vi "Main.vi"(10 "JQMHStartup":refnum<class "RQMHStartup.lvclass">, 11 "NewTemplate in":refnum<class "CRON.lvclass">) -> ()   [LabVIEW 2024, in "CRON.lvclass"]
uses:
  CRON.lvclass
  C:/DevOps/CORTEX/JQMH/RQMHCore/ModuleCore/RQMHModule.lvclass
  RQMHCore/Startup/RQMHStartup.lvclass
  <vilib>/LabVIEW Open Source Project/Cron Scheduler/Cron/Cron.lvclass
  RQMHCore/ModQueue/RQMHMessageQueue.lvclass/RQMHMessageQueue.ctl
  RQMHCore/ModuleCore/InitialiseReplyArgs.ctl
  <vilib>/Utility/miscctls.llb/LVPointTypeDef.ctl
  RQMHCore/ModuleCore/RQMHModule.lvclass/RQMHModule.ctl
  Do Something ReplyArgs.ctl
  Do Something Args.ctl
  RQMHCore/ModuleCore/Read ModuleName.vi
  RQMHCore/ModuleCore/Read External Start.vi
  RQMHCore/ModQueue/Delacor_lib_QMH_Enqueue Message (Single).vi
  RQMHCore/ModQueue/RQMHMessageQueue.lvclass
  RQMHCore/ModuleCore/RQMHModule.lvclass
  RQMHCore/Shared/RQMHShared.lvlib
  <vilib>/LabVIEW Open Source Project/Cron Scheduler/openCron.lvlib
panel:
  out "error out":errorcluster
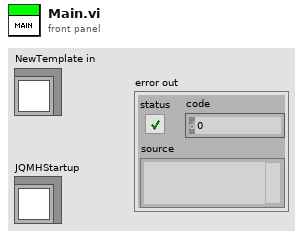
[diagram p1: front panel]
types:
  T1 = typedef "CRON.lvclass/Request Events--cluster.ctl" = cluster{"Do Something":refnum<user-event>, "Set Schedule":refnum<user-event>, "Arm":refnum<user-event>}
  T2 = cluster{"Stop Module":refnum<user-event>, "Requests":T1}
  T3 = typedef "LVPointTypeDef.ctl" = cluster{"Horizontal":i16, "Vertical":i16}
  T4 = enum32{"Invalid", "Standard", "Closed", "Hidden", "Minimized", "Maximized"}
  T5 = typedef "RQMHModule.lvclass/InitialiseReplyArgs.ctl" = cluster{"Did Init?":bool}
  T6 = typedef "CRON.lvclass/Do Something Args.ctl" = cluster{"Msg":string}
  T7 = typedef "CRON.lvclass/Do Something ReplyArgs.ctl" = cluster{"Value":dbl, "Boolean":bool}
  T8 = typedef "RQMHModule.lvclass/Reply.ctl" = cluster{"Expects Reply":bool, "Reply":refnum<notifier>}
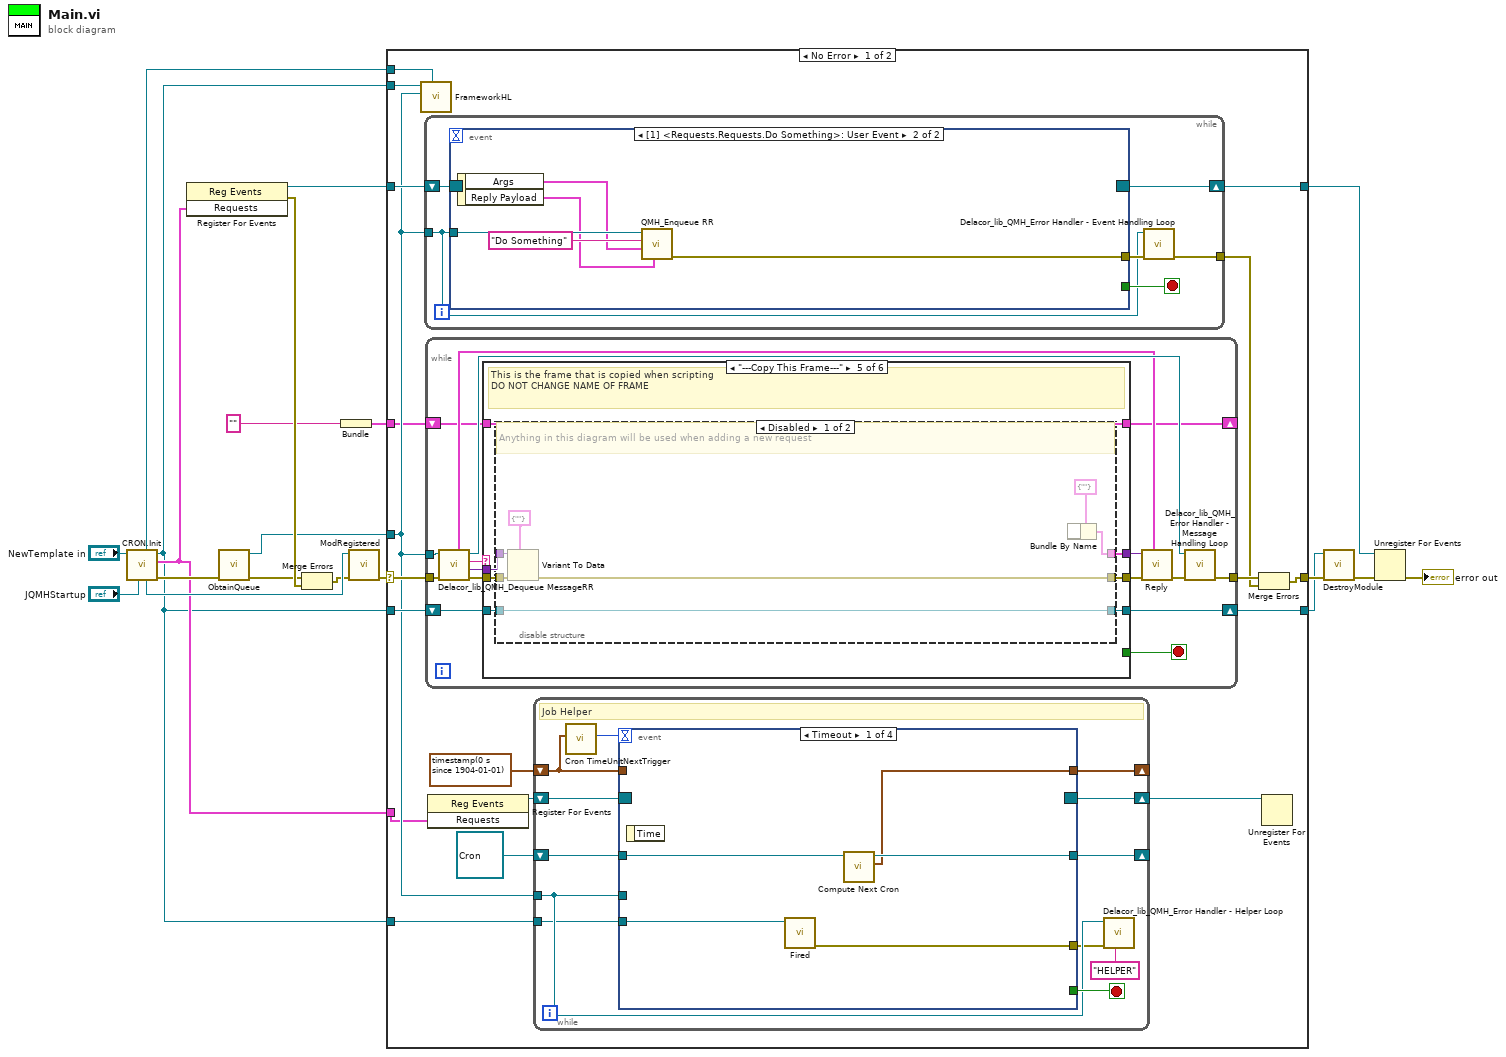
[diagram p0: block diagram]
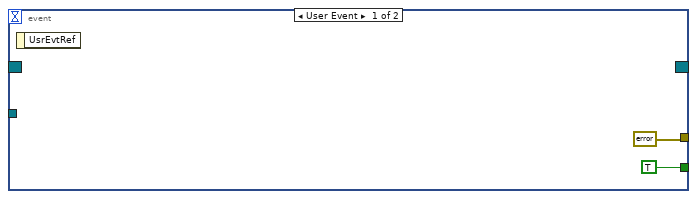
[diagram p2: hidden frame]
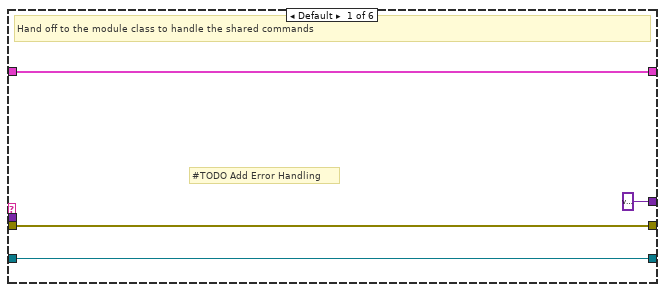
[diagram p3: hidden frame]
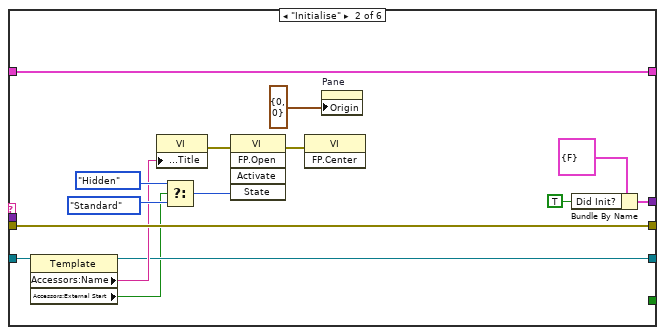
[diagram p4: hidden frame]
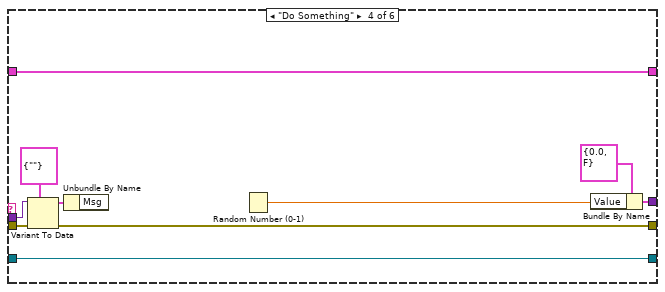
[diagram p6: hidden frame]
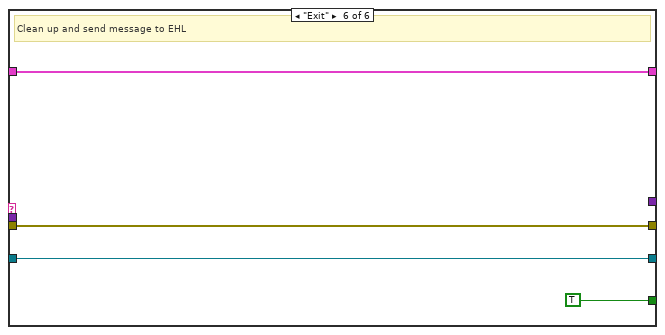
[diagram p8: hidden frame]
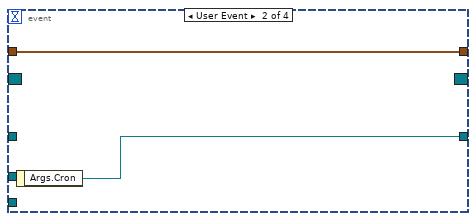
[diagram p9: hidden frame]
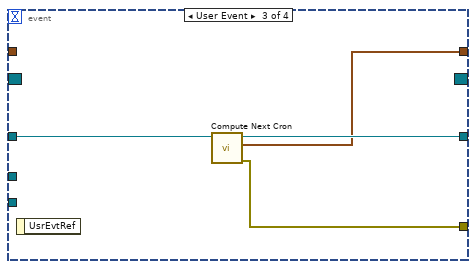
[diagram p10: hidden frame]
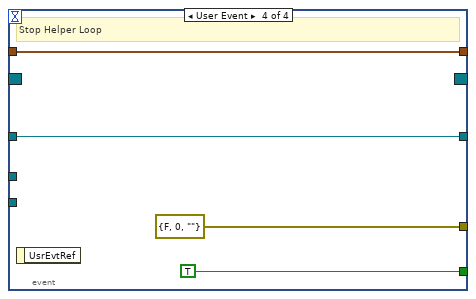
[diagram p11: hidden frame]
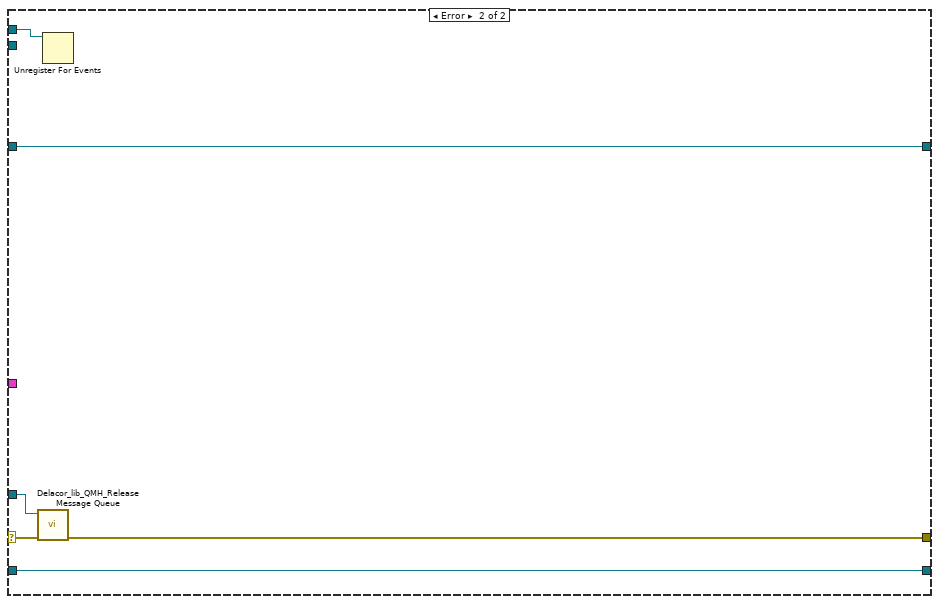
[diagram p12: hidden frame]
diagram:
  n1 = call "CRON.Init.vi"("JQMHStartup in"="JQMHStartup", "NewTemplate in"="NewTemplate in") -> ("error out"=w13:errorcluster, "Requests"=w2:T2, "NewTemplate out"=w1:refnum<class "CRON.lvclass">, "JQMHStartup out"=w11:refnum<class "RQMHStartup.lvclass">, "StandardRequests"=w7:refnum<event-registration>)  [unwired: 3 in, 2 out]
  n2 = register-events(w2) -> (reference out=w6:refnum<event-registration>, error out=w20:errorcluster)  [unwired: 2 in]
  n3 = call "ObtainQueue.vi"("error in"=w13) -> ("error out"=w12:errorcluster, "Message Queue"=w8:refnum<class "RQMHMessageQueue.lvclass">)  [unwired: 9 in]
  n4 = Merge Errors(w12, w20) -> (w9:errorcluster)
  n5 = Bundle("") -> (w4:cluster{string})  [unwired: 1 in]
  n6 = call "ModRegistered.vi"("error in (no error)"=w9, "JQMHStartup in"=w11) -> ("error out"=w10:errorcluster)  [unwired: 9 in]
  n7 = case "RQMH_MAIN" shown="No Error" w10 {
    selector: w10 -> [w35 w150]
    tunnel: w1 -> [w38 w149]
    tunnel: [w37 w152] -> w19
    tunnel: w6 -> [w36 w152]
    tunnel: w8 -> [w29 w151]
    tunnel: [w34 w149] -> w5
    tunnel: [w31 w148] -> w16
    tunnel: w1 -> [w30 _]
    tunnel: w7 -> [w28 w147]
    tunnel: w4 -> [w27 _]
    tunnel: w2 -> [w26 _]
    tunnel: w1 -> [w25 _]
    frame No Error {
      n8 = call-dynamic "FrameworkHL.vi"("StandardRequests"=w28, "Message Queue"=w29, "JQMHModule in"=w30) -> ()  [unwired: 9 in]
      n9 = while {
        shift-right: [w44] -> w37
        shift-left: w36 -> [w39]
        tunnel: w29 -> [w40]
        tunnel: [w41] -> w32
        stop <- w43 stop-if-true
        n10 = event "RQMH_EVENT_MAIN" shown="[1] <Requests.Requests.Do Something>: User Event" {
          selector: w39 -> [_ _]
          dyn-events: [_ _] -> w44
          timeout: _ -> [_ _]
          tunnel: [TRUE _] -> w43
          tunnel: w40 -> [_ w51]
          tunnel: [errorcluster {"status"=FALSE, "code"=0, "source"=""} ("error out") w48] -> w42
          event User Event {
            n11 = event-data() -> ()  [unwired: 1 in, 1 out]
          }
          event User Event {
            n12 = event-data() -> ("Args"=w49:T6, "Reply Payload"=w47:T8)  [unwired: 1 in]
            n13 = call "QMH_Enqueue RR.vi"("Reply"=w47, "Message Data"=w49, "Message"="Do Something", "Message Queue in"=w51) -> ("error out"=w48:errorcluster)  [unwired: 6 in, 1 out]
          }
        }
        n14 = call-dynamic "Delacor_lib_QMH_Error Handler - Event Handling Loop.vi"("error in"=w42, "Message Queue in"=w40) -> ("dup error in"=w41:errorcluster)  [unwired: 8 in, 1 out]
      }
      n15 = while {
        tunnel: w29 -> [w62]
        tunnel: w35 -> [w61]
        shift-right: [w64] -> w34
        shift-left: w38 -> [w65]
        tunnel: [w63] -> w33
        shift-right: [w52] -> _
        shift-left: w27 -> [w53]
        stop <- w67 stop-if-true
        n16 = call-dynamic "Delacor_lib_QMH_Dequeue MessageRR.vi"("error in"=w61, "Message Queue in"=w62) -> ("error out"=w60:errorcluster, "Message Data"=w58:variant, "Message"=w59:string, "Message Queue out"=w66:refnum<class "RQMHMessageQueue.lvclass">, "Reply"=w54:T8)  [unwired: 5 in]
        n17 = case "RQMH_MESSAGE_CASES" shown="Default" w59 {
          tunnel: [_ _ _ _ _ TRUE] -> w67
          tunnel: w65 -> [w70 w74 w88 w99 w104 w118]
          tunnel: w58 -> [_ _ _ w95 w102 _]
          tunnel: w60 -> [w71 w86 w89 w94 w106 w117]
          tunnel: [w71 w86 w89 w93 w105 w117] -> w57
          tunnel: [w70 w75 w88 w99 w103 w118] -> w64
          tunnel: [variant w85 _ w98 w101 _] -> w55
          tunnel: w53 -> [w68 w72 w87 w90 w100 w116]
          tunnel: [w68 w72 w87 w90 w100 w116] -> w52
          frame Default {
            # "#TODO Add Error Handling"
            # "Hand off to the module class to handle the shared commands"
          }
          frame "Initialise" {
            n18 = property class="Template"(reference=w74) -> (reference out=w75:refnum<class "CRON.lvclass">, "Accessors:Name"=w76:string, "Accessors:External Start"=w73:bool)  [unwired: 1 in, 1 out]
            n19 = property on="Property Node" class="VI"("Front Panel.Title"=w76) -> (error out=w83:errorcluster)  [unwired: 2 in, 1 out]
            n20 = Select(t=T4."Hidden" ("State"), s=w73, f=T4."Standard" ("State")) -> (s? t:f=w79:T4)
            n21 = invoke on="Invoke Node" class="VI" method="FP.Open"(error in=w83, "State"=w79) -> (error out=w82:errorcluster)  [unwired: 3 in, 4 out]
            n22 = invoke on="Invoke Node" class="VI" method="FP.Center"(error in=w82) -> ()  [unwired: 2 in, 3 out]
            n23 = property on="Pane" class="Pane"("Origin"=T3 {"Horizontal"=0, "Vertical"=0}) -> ()  [unwired: 2 in, 2 out]
            n24 = Bundle By Name(cluster=T5 {"Did Init?"=FALSE} ("Args"), "Did Init?"=TRUE) -> (w85:T5)
          }
          frame "---Module Specific---" {
          }
          frame "Do Something" {
            n25 = Variant To Data(error in=w94, type=T6 {"Msg"=""} ("Do Something Args"), Variant=w95) -> (data=w91:T6, error out=w93:errorcluster)
            n26 = Unbundle By Name(w91) -> ()  [unwired: 1 out]
            n27 = Random Number (0-1)() -> (number: 0 to 1=w96:dbl)
            n28 = Bundle By Name(cluster=T7 {"Value"=0.0, "Boolean"=FALSE}, "Value"=w96) -> (w98:T7)
          }
          frame "---Copy This Frame---" {
            # "This is the frame that is copied when scripting\nDO NOT CHANGE NAME OF FRAME"
            n29 = disable-structure shown="Disabled" {
              disable-tunnel: w106 -> [w110 w115]
              disable-tunnel: [w111 w115] -> w105
              disable-tunnel: w104 -> [w113 w114]
              disable-tunnel: [w113 w114] -> w103
              disable-tunnel: w102 -> [w112 _]
              disable-tunnel: [w108 _] -> w101
              frame Disabled {
                # "Anything in this diagram will be used when adding a new request"
                n30 = Variant To Data(error in=w110, type=cluster{string} {""} ("RQMH_MHL_MSG_PL"), Variant=w112) -> (error out=w111:errorcluster)  [unwired: 1 out]
                n31 = Bundle By Name(cluster=cluster{string} {""} ("RQMH_MHL_REPLY_PL")) -> (w108:cluster{string})  [unwired: 1 in]
              }
              frame Enabled {
              }
            }
          }
          frame "Exit" {
            # "Clean up and send message to EHL"
          }
        }
        n32 = call "Reply.vi"("Reply"=w54, "error in (no error)"=w57, "ReplyPayload"=w55) -> ("error out"=w56:errorcluster)  [unwired: 8 in]
        n33 = call-dynamic "Delacor_lib_QMH_Error Handler - Message Handling Loop.vi"("error in"=w56, "Message Queue in"=w66) -> ("dup error in"=w63:errorcluster)  [unwired: 8 in, 1 out]
      }
      n34 = register-events ("DQMH_HELPER_REGFOREVENTS")(w26) -> (reference out=w24:refnum<event-registration>)  [unwired: 2 in, 1 out]
      n35 = while "RQMH_HELPER_LOOP" {
        shift-right: [w131] -> _
        shift-left: timestamp(0 s since 1904-01-01) ("Next Occurence") -> [w121]
        shift-right: [w129] -> w23
        shift-left: w24 -> [w130]
        tunnel: w29 -> [w127]
        tunnel: w25 -> [w122]
        shift-right: [w123] -> _
        shift-left: refnum<class "Cron.lvclass"> refnum ("Cron in") -> [w124]
        stop <- w128 stop-if-true
        # "Job Helper"
        n36 = call <vilib>:"Cron TimeUnitNextTrigger.vi"("Next Occurence"=w121) -> ("next event (ms)"=w120:i32)  [unwired: 10 in]
        n37 = event "RQMH_HELPER_EVENT_STRUCTURE" shown="[0] Timeout" {
          selector: w130 -> [_ _ _ _]
          dyn-events: [_ _ _ _] -> w129
          timeout: w120 -> [_ _ _ _]
          tunnel: w121 -> [_ w138 _ w143]
          tunnel: [w132 w138 w140 w143] -> w131
          tunnel: [_ _ _ TRUE] -> w128
          tunnel: [w135 _ w139 errorcluster {"status"=FALSE, "code"=0, "source"=""} ("error constant")] -> w125
          tunnel: w127 -> [_ _ _ _]
          tunnel: w124 -> [w133 _ w141 w144]
          tunnel: [w134 w137 w142 w144] -> w123
          tunnel: w122 -> [w136 _ _ _]
          event Timeout {
            n38 = event-data() -> ()  [unwired: 1 in, 1 out]
            n39 = call "Fired.vi"("module in"=w136) -> ("error out"=w135:errorcluster)  [unwired: 9 in, 1 out]
            n40 = call <vilib>:"Compute Next Cron.vi"("Cron in"=w133) -> ("Next Occurence"=w132:timestamp, "Cron out"=w134:refnum<class "Cron.lvclass">)  [unwired: 7 in, 2 out]
          }
          event User Event {
            n41 = event-data() -> ("Args.Cron"=w137:refnum<class "Cron.lvclass">)  [unwired: 1 in]
          }
          event User Event {
            n42 = event-data() -> ()  [unwired: 1 in, 1 out]
            n43 = call <vilib>:"Compute Next Cron.vi"("Cron in"=w141) -> ("error out"=w139:errorcluster, "Next Occurence"=w140:timestamp, "Cron out"=w142:refnum<class "Cron.lvclass">)  [unwired: 7 in, 1 out]
          }
          event User Event {
            # "Stop Helper Loop"
            n44 = event-data() -> ()  [unwired: 1 in, 1 out]
          }
        }
        n45 = call-dynamic "Delacor_lib_QMH_Error Handler - Helper Loop.vi"("HelperName"="HELPER" ("RQMH_HELPER_LOOP_NAME"), "error in"=w125, "Message Queue in"=w127) -> ()  [unwired: 7 in, 2 out]
      }
      n46 = Merge Errors(w33, w32) -> (w31:errorcluster)
      n47 = Unregister For Events(event registration refnum=w23) -> ()  [unwired: 1 in, 1 out]
    }
    frame Error {
      n48 = call-dynamic "Delacor_lib_QMH_Release Message Queue.vi"("error in"=w150, "Message Queue"=w151) -> ("error out"=w148:errorcluster)  [unwired: 9 in]
      n49 = Unregister For Events(event registration refnum=w147) -> ()  [unwired: 1 in, 1 out]
    }
  }
  n50 = call "DestroyModule.vi"("error in (no error)"=w16, "JQMHModule in"=w5) -> ("error out"=w18:errorcluster)  [unwired: 9 in]
  n51 = Unregister For Events(event registration refnum=w19, error in=w18) -> (error out=→"error out":errorcluster)
